vi "mxwScript_Cmnd2Str_setUniquificationObjects.vi"(8 "error in (no error)":errorcluster, 11 "data":variant) -> (0 "error out":errorcluster, 3 "outputString":string)   [LabVIEW 2017]
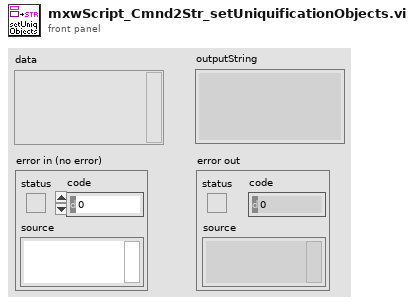
[diagram p1: front panel]
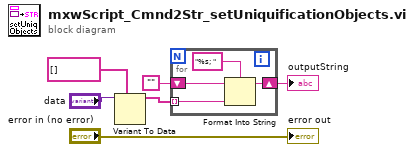
[diagram p0: block diagram]
diagram:
  n1 = Variant To Data(type=string[] [], Variant="data") -> (data=w4:string[])  [unwired: 1 in, 1 out]
  n2 = for {
    tunnel: w4 -> [w7] mode=indexing
    shift-right: [w9] -> w2
    shift-left: "" -> [w8]
    n3 = Format Into String(format string="%s; ", initial string=w8, w7) -> (resulting string=w9:string)  [unwired: 1 in, 1 out]
  }
  "outputString" <- w2
  "error out" <- "error in (no error)"
